vi "Send Message.vi"(4 "timeout in ms (100)":i32=100, 6 "Message ID":i32, 8 "error in (no error)":errorcluster, 9 "Data":variant, 10 "Command":string, 11 "RemoteControl.ZMQ in":refnum<class "RemoteControl.ZMQ.lvclass">) -> (0 "error out":errorcluster, 2 "ACK":string, 3 "RemoteControl.ZMQ out":refnum<class "RemoteControl.ZMQ.lvclass">)   [LabVIEW 2019, in "RemoteControl.ZMQ.lvclass"]
uses:
  RemoteControl.ZMQ.lvclass
  <vilib>/addons/zeromq/zmq_socket.lvclass
  RemoteControl/Typedefs/Message--Cluster.ctl
  RemoteControl/RemoteControl.lvclass
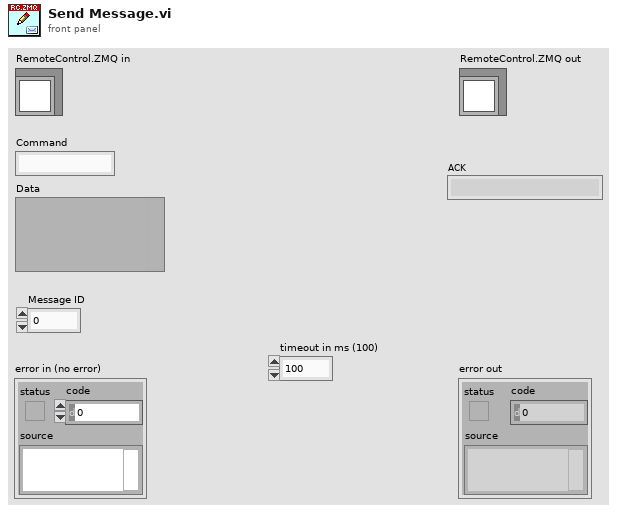
[diagram p1: front panel]
types:
  T1 = typedef "RemoteControl.lvclass/Message--Cluster.ctl" = cluster{"Command":string, "Data":variant, "Message ID":i32}
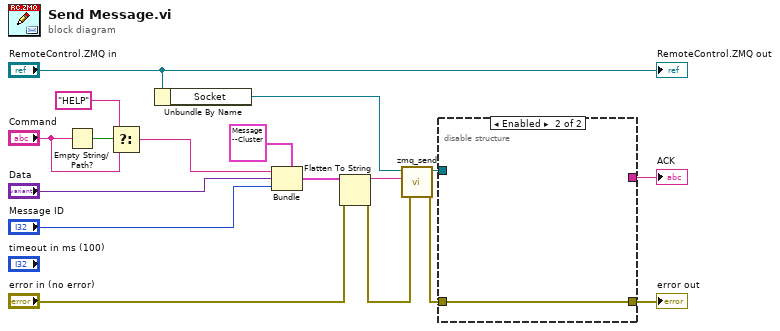
[diagram p0: block diagram]
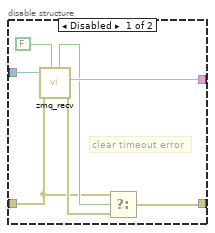
[diagram p2: hidden frame]
diagram:
  n1 = Empty String/Path?(string/path="Command") -> (empty?=w11:bool)
  n2 = Select(t="HELP", s=w11, f="Command") -> (s? t:f=w14:string)
  n3 = Unbundle By Name("RemoteControl.ZMQ in") -> ("Socket"=w3:refnum<class "zmq_socket.lvclass">)
  n4 = Bundle(cluster=T1 {"Command"="", "Data"=variant, "Message ID"=0} ("Message"), "Command"=w14, "Data"="Data", "Message ID"="Message ID") -> (w4:T1)
  n5 = Flatten To String(anything=w4, error in (no error)="error in (no error)") -> (data string=w7:string, error out=w5:errorcluster)  [unwired: 2 in, 1 out]
  n6 = call <vilib>:"zmq_send.vi"("error in"=w5, "data"=w7, "socket in"=w3) -> ("error out"=w1:errorcluster, "socket out"=w9:refnum<class "zmq_socket.lvclass">)  [unwired: 4 in]
  n7 = disable-structure shown="Enabled" {
    disable-tunnel: w9 -> [w24 _]
    disable-tunnel: [w23 _] -> w8
    disable-tunnel: [w19 w25] -> w2
    disable-tunnel: w1 -> [w18 w25]
    frame Disabled {
      # "clear timeout error"
      n8 = call <vilib>:"zmq_recv.vi"("no block? (F)"=FALSE, "error in"=w18, "socket in"=w24) -> ("error out"=w20:errorcluster, "data"=w23:string, "timeout?"=w21:bool)  [unwired: 2 in, 2 out]
      n9 = Select(t=w18, s=w21, f=w20) -> (s? t:f=w19:errorcluster)
    }
    frame Enabled {
    }
  }
  "error out" <- w2
  "ACK" <- w8
  "RemoteControl.ZMQ out" <- "RemoteControl.ZMQ in"
